vi "read FGV.vi"() -> ()   [LabVIEW 2019]
panel:
  in  "stop":bool
  out "Array":dbl[](array[numeric])
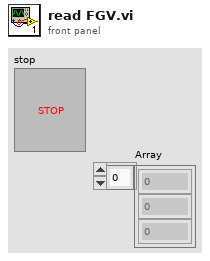
[diagram p1: front panel]
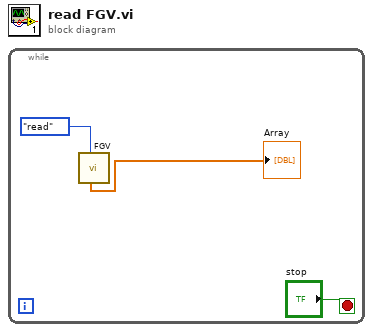
[diagram p0: block diagram]
diagram:
  n1 = while {
    stop <- "stop" stop-if-true
    n2 = call "FGV.vi"("action"=enum16{"read", "write"}."read") -> ("read"=→"Array":dbl[])  [unwired: 10 in]
  }
